vi "Remove.vi"(8 "error in (no error)":errorcluster, 11 "LV MDI in":refnum<class "LV MDI.lvclass">) -> (0 "error out":errorcluster, 3 "LV MDI out":refnum<class "LV MDI.lvclass">)   [LabVIEW 2016, in "LV MDI.lvclass"]
uses:
  LV MDI.lvclass
  LV MDI.lvclass/LV MDI.ctl
  user32.dll
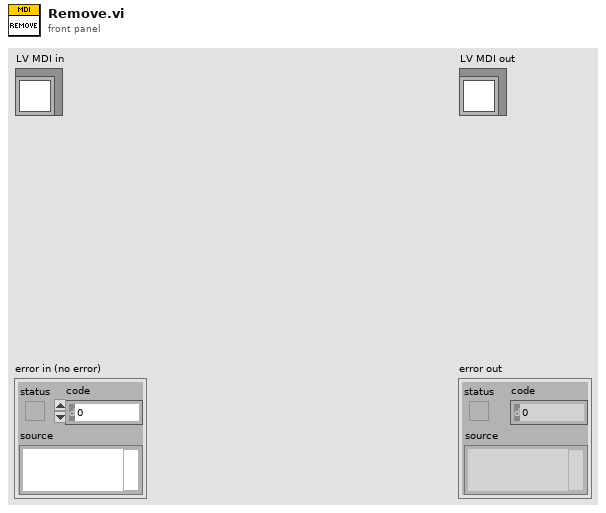
[diagram p1: front panel]
types:
  T1 = typedef "LV MDI.lvclass/Window Data.ctl" = cluster{"Child hWnd":u32, "UID":string, "vi reference":refnum<vi>, "Name":string}
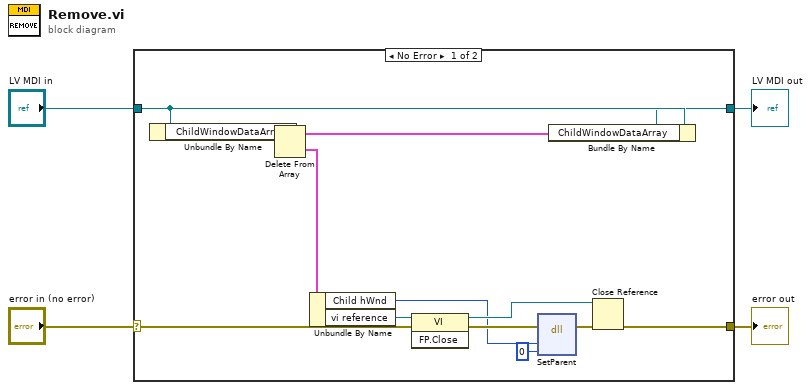
[diagram p0: block diagram]
diagram:
  n1 = case shown="No Error" "error in (no error)" {
    selector: "error in (no error)" -> [w17 w19]
    tunnel: [w10 w19] -> w3
    tunnel: [w13 w18] -> w1
    tunnel: "LV MDI in" -> [w14 w18]
    frame No Error {
      n2 = Unbundle By Name(w14) -> ("ChildWindowDataArray"=w16:T1[])
      n3 = Delete From Array(array=w16) -> (deleted portion=w15:T1, array with subset deleted=w12:T1[])  [unwired: 2 in]
      n4 = Unbundle By Name(w15) -> ("Child hWnd"=w7:u32, "vi reference"=w5:refnum<vi>)
      n5 = invoke class="VI" method="FP.Close"(reference=w5, error in=w17) -> (reference out=w9:refnum<vi>, error out=w11:errorcluster)  [unwired: 1 in, 1 out]
      n6 = dll-call lib="user32.dll" fn="SetParent"(error in=w11, "Child"=w7, "NewParent"=0) -> (error out=w8:errorcluster)  [unwired: 5 in, 1 out]
      n7 = Bundle By Name(cluster=w14, "ChildWindowDataArray"=w12) -> (w13:refnum<class "LV MDI.lvclass">)
      n8 = Close Reference(reference=w9, error in (no error)=w8) -> (error out=w10:errorcluster)
    }
    frame Error {
    }
  }
  "error out" <- w3
  "LV MDI out" <- w1
